vi "waitForNewResults.vi"(8 "error in (no error)":errorcluster, 11 "Instrument.Lockin in":refnum<class "Instrument.Lockin.lvclass">) -> (0 "error out":errorcluster, 2 "Results":dbl[][](array[numeric]), 3 "Instrument.Lockin out":refnum<class "Instrument.Lockin.lvclass">)   [LabVIEW 2016, in "Instrument.Lockin.lvclass"]
uses:
  Instrument.Lockin.lvclass
  <vilib>/Utility/error.llb/Error Cluster From Error Code.vi
  <vilib>/ErrorRing/Error Ring.xnode
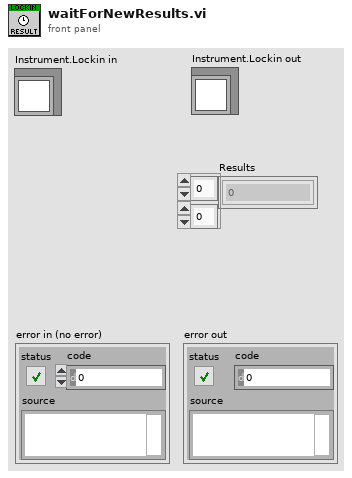
[diagram p1: front panel]
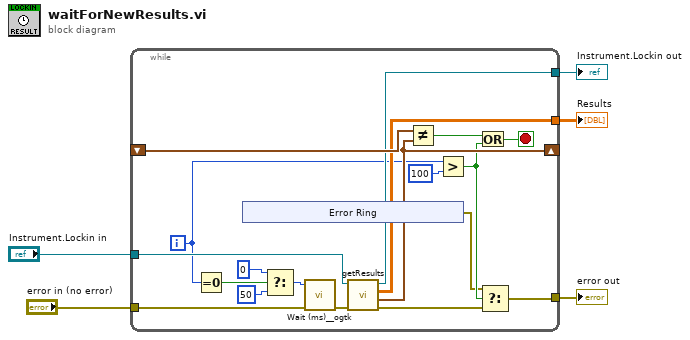
[diagram p0: block diagram]
diagram:
  n1 = while {
    shift-right: [w21] -> _
    shift-left: _ -> [w23]
    tunnel: "error in (no error)" -> [w24]
    tunnel: [w11] -> w5
    tunnel: [w20] -> w3
    tunnel: "Instrument.Lockin in" -> [w19]
    tunnel: [w18] -> w1
    i -> [w10]
    stop <- w16 stop-if-true
    n2 = Equal To 0?(x=w10) -> (x = 0?=w9:bool)
    n3 = xnode "Error Ring"() -> ("error out"=w13:errorcluster)
    n4 = Select(t=u32 0, s=w9, f=u32 50 ("milliseconds to wait")) -> (s? t:f=w7:u32)
    n5 = call <userlib>:"Wait (ms)__ogtk.vi"("error in (no error)"=w24, "milliseconds to wait"=w7) -> ("error out"=w22:errorcluster)  [unwired: 8 in, 1 out]
    n6 = call "getResults.vi"("error in (no error)"=w22, "Instrument.Lockin in"=w19) -> ("error out"=w12:errorcluster, "Time Stamp"=w21:timestamp, "Results"=w20:dbl[][], "Instrument.Lockin out"=w18:refnum<class "Instrument.Lockin.lvclass">)  [unwired: 6 in]
    n7 = Not Equal?(x=w23, y=w21) -> (x != y?=w17:bool)
    n8 = Greater?(x=w10, y=100) -> (0:w14:bool)
    n9 = Or(x=w17, y=w14) -> (x .or. y?=w16:bool)
    n10 = Select(t=w13, s=w14, f=w12) -> (s? t:f=w11:errorcluster)
  }
  "error out" <- w5
  "Results" <- w3
  "Instrument.Lockin out" <- w1
